vi "Modify Constructor.vi"(8 "error in (no error)":errorcluster, 11 "QControl Creation in":refnum<class "QControl Creation.lvclass">) -> (0 "error out":errorcluster, 3 "QControl Creation out":refnum<class "QControl Creation.lvclass">)   [LabVIEW 2020, in "QControl Creation.lvclass"]
doc: "<b> </b> <b> </b>\n©2016 Q Software Innovations, LLC (QSI)\nwritten by Quentin Alldredge\nproduced in LabVIEW 2015\n\nsupport@qsoftwareinnovations.com\nwww.qsoftwareinnovations.com\n\nAll rights reserved.\n\nRedistribution and use in source and binary forms, with or without modification, are permitted provided that the following conditions are met:\n\n * Redistributions of source code must retain the above copyright notice, this list of conditions and the following disclaimer.\n * Redistributions in binary form must reproduce the above copyright notice, this list of conditions and the following disclaimer in the documentation and/or other materials provided with the distribution.\n * Neither the name of Q Software Innovations, LLC. nor the names of its contributors may be used to endorse or promote products derived from this software without specific prior written permission.\n\nTHIS SOFTWARE IS PROVIDED BY THE COPYRIGHT HOLDERS AND CONTRIBUTORS \"AS IS\" AND ANY EXPRESS OR IMPLIED WARRANTIES, INCLUDING, BUT NOT LIMITED TO, THE IMPLIED WARRANTIES OF MERCHANTABILITY AND FITNESS FOR A PARTICULAR PURPOSE ARE DISCLAIMED. IN NO EVENT SHALL THE COPYRIGHT OWNER OR CONTRIBUTORS BE LIABLE FOR ANY DIRECT, INDIRECT, INCIDENTAL, SPECIAL, EXEMPLARY, OR CONSEQUENTIAL DAMAGES (INCLUDING, BUT NOT LIMITED TO, PROCUREMENT OF SUBSTITUTE GOODS OR SERVICES; LOSS OF USE, DATA, OR PROFITS; OR BUSINESS INTERRUPTION) HOWEVER CAUSED AND ON ANY THEORY OF LIABILITY, WHETHER IN CONTRACT, STRICT LIABILITY, OR TORT (INCLUDING NEGLIGENCE OR OTHERWISE) ARISING IN ANY WAY OUT OF THE USE OF THIS SOFTWARE, EVEN IF ADVISED OF THE POSSIBILITY OF SUCH DAMAGE."
uses:
  QControl Creation.lvclass
  QControl Creation.lvclass/QControl Creation.ctl
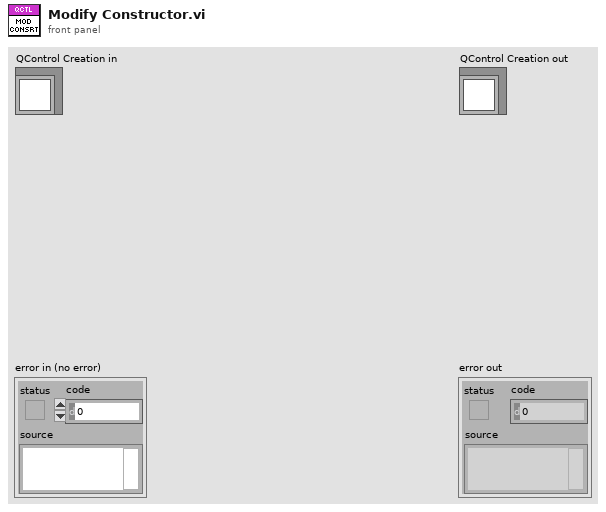
[diagram p1: front panel]
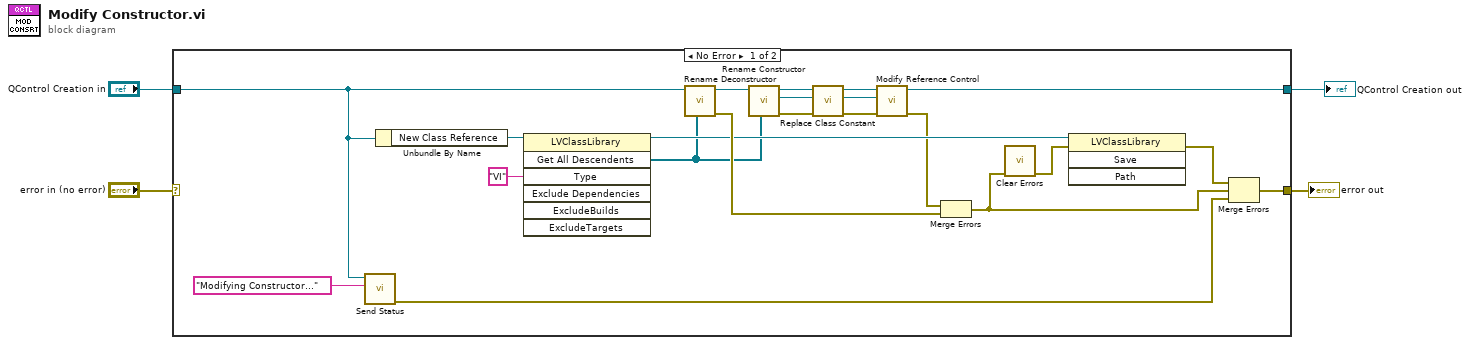
[diagram p0: block diagram]
diagram:
  n1 = case shown="No Error" "error in (no error)" {
    selector: "error in (no error)" -> [_ w27]
    tunnel: [w15 w27] -> w3
    tunnel: "QControl Creation in" -> [w7 w26]
    tunnel: [w8 w26] -> w1
    frame No Error {
      n2 = call "Send Status.vi"("Status"="Modifying Constructor..." ("Add Item"), "QControl Creation in"=w7) -> ("error out (dup)"=w14:errorcluster)  [unwired: 8 in, 1 out]
      n3 = Unbundle By Name(w7) -> ("New Class Reference"=w25:refnum<vi>)
      n4 = invoke class="LVClassLibrary" method="Get All Descendents"(reference=w25, "Type"="VI") -> (reference out=w20:refnum<vi>, "All Descendents"=w5:refnum<vi>[])  [unwired: 5 in, 5 out]
      n5 = call "Rename Deconstructor.vi"("All Descendents"=w5, "QControl Creation in"=w7) -> ("error out"=w22:errorcluster, "QControl Creation out"=w6:refnum<class "QControl Creation.lvclass">)  [unwired: 8 in]
      n6 = call "Rename Constructor.vi"("All Descendents"=w5, "QControl Creation in"=w6) -> ("error out"=w21:errorcluster, "Constructor Method VI out"=w10:refnum<vi>, "QControl Creation out"=w9:refnum<class "QControl Creation.lvclass">)  [unwired: 7 in]
      n7 = call "Replace Class Constant.vi"("error in (no error)"=w21, "Constructor Method VI in"=w10, "QControl Creation in"=w9) -> ("error out"=w13:errorcluster, "Constructor Method VI (dup)"=w12:refnum<vi>, "QControl Creation (dup)"=w11:refnum<class "QControl Creation.lvclass">)  [unwired: 6 in]
      n8 = call "Modify Reference Control.vi"("error in (no error)"=w13, "Constructor Method VI in"=w12, "QControl Creation in"=w11) -> ("error out"=w19:errorcluster, "QControl Creation (dup)"=w8:refnum<class "QControl Creation.lvclass">)  [unwired: 7 in]
      n9 = Merge Errors(w19, w22) -> (w17:errorcluster)
      n10 = call <vilib>:"Clear Errors.vi"("error in (no error)"=w17) -> ("error out"=w18:errorcluster)  [unwired: 5 in, 1 out]
      n11 = invoke class="LVClassLibrary" method="Save"(reference=w20, error in=w18) -> (error out=w16:errorcluster)  [unwired: 2 in, 3 out]
      n12 = Merge Errors(w16, w17, w14) -> (w15:errorcluster)
    }
    frame Error {
    }
  }
  "error out" <- w3
  "QControl Creation out" <- w1
